vi "API Demo.vi"() -> ()   [LabVIEW 2020]
uses:
  Framework/Test Case/LUnit Test Case.lvclass
  Framework/Result Classes/Method Result/Method Result.lvclass/Method Result.ctl
  Framework/Result Classes/Test Case Result/Test Case Result.lvclass/Test Case Result.ctl
  Framework/Result Classes/Test Suite Result/Test Suite Result.lvclass/Test Suite Result.ctl
  Framework/Result Classes/Test Case Result/Private/SubVIs/Merge Status.vi
  Framework/Execution API/Execution API.lvclass
  Framework/Result Classes/Method Result/Method Result.lvclass
  Framework/Result Classes/Test Case Result/Test Case Result.lvclass
  Framework/Result Classes/Test Suite Result/Test Suite Result.lvclass
panel:
  in  "Tab Control":enum32{"Path", "Test Case", "App Instance"}(tab)
  in  "Project or Class Path":path
  in  "Class path":path
  out "error out":errorcluster
  in  "error in":errorcluster
  in  "Stop":bool
  out "Status":string
  # "1. Select which method you want to use for finding tests to run from the API by choosing a tab in the tab control.\n2. Fill in the path to the test to run. \n3. Run this VI."
  # "Enter the path to a test case class, lvlib or a project containing the test cases."
  # "Execute all tests found in the current application instance"
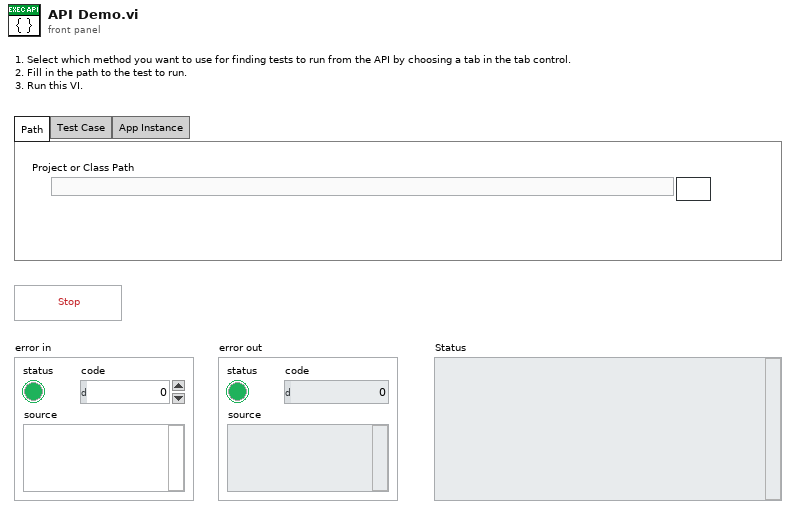
[diagram p1: front panel]
types:
  T1 = cluster{"Event Registration Refnum":refnum<event-registration>, "Event Registration Refnum":refnum<event-registration>}
  T2 = typedef "Assertion Result.lvclass/Status.ctl" = enum16{"Pass", "Fail", "Error", "Skipped", "Setup Error", "Broken", "Teardown Error"}
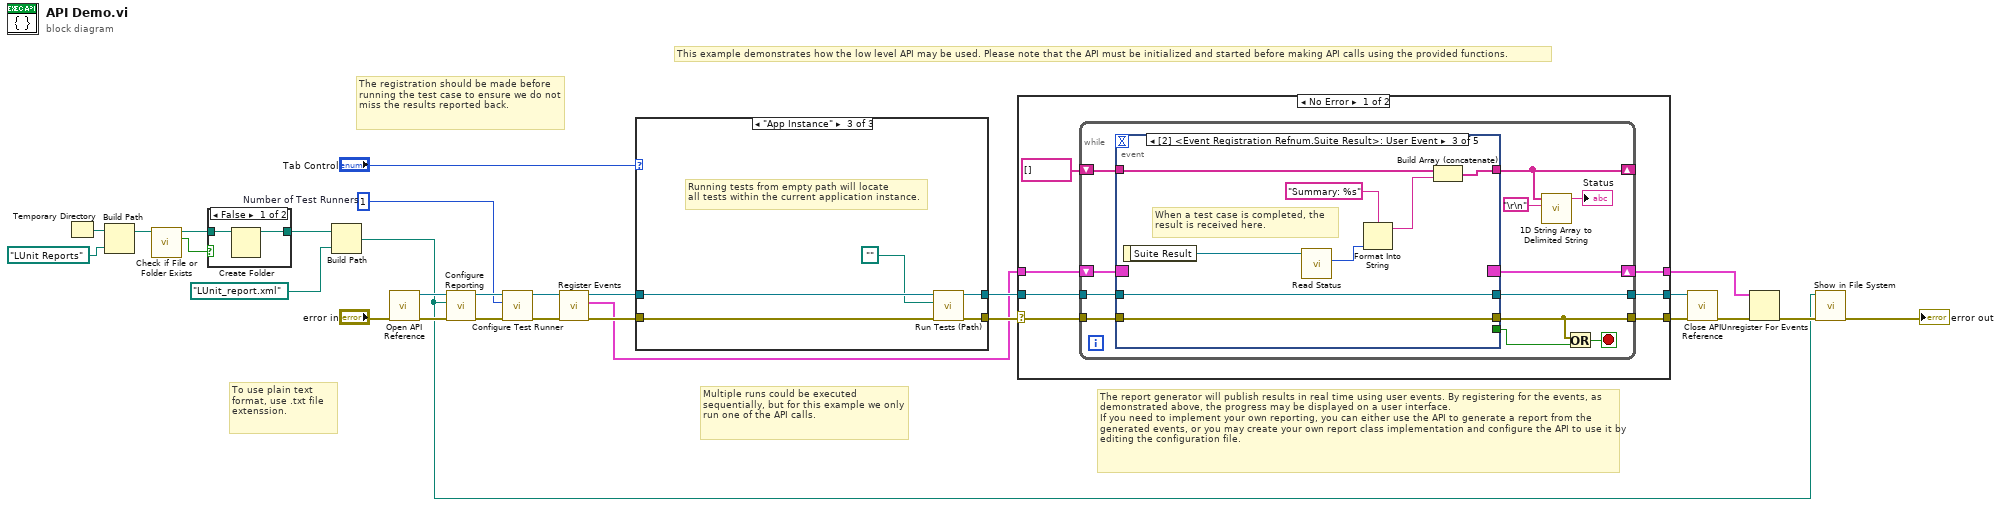
[diagram p0: block diagram]
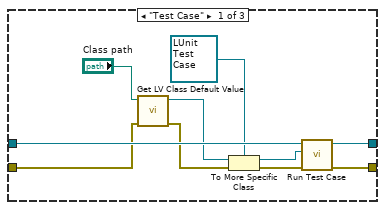
[diagram p3: hidden frame]
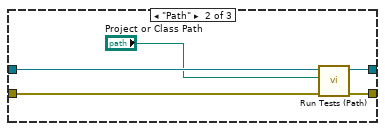
[diagram p4: hidden frame]
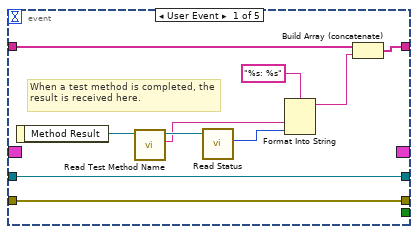
[diagram p5: hidden frame]
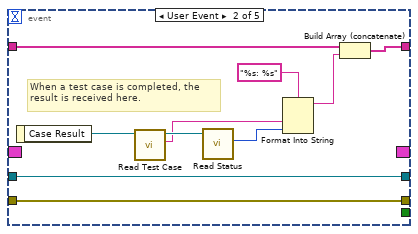
[diagram p6: hidden frame]
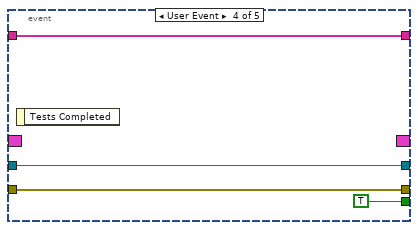
[diagram p7: hidden frame]
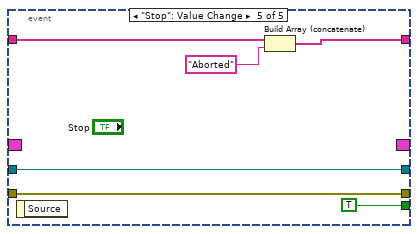
[diagram p8: hidden frame]
diagram:
  w11 = 1  # Number of Test Runners
  # "To use plain text format, use .txt file extenssion."
  # "The registration should be made before running the test case to ensure we do not miss the results reported back."
  # "The report generator will publish results in real time using user events. By registering for the events, as demonstrated above, the progress may be displayed on a user interface. \nIf you need to implement your own reporting, you can either use the API to generate a report from the generated events, or you may create your own report class implementation and configure the API to use it by editing the configuration file."
  # "This example demonstrates how the low level API may be used. Please note that the API must be initialized and started before making API calls using the provided functions."
  # "Multiple runs could be executed sequentially, but for this example we only run one of the API calls."
  n1 = Temporary Directory() -> (w5:path)
  n2 = Build Path(base path=w5, name or relative path=path "LUnit Reports") -> (appended path=w6:path)
  n3 = call <vilib>:"Check if File or Folder Exists.vi"("path"=w6) -> ("file or folder exists?"=w2:bool, "dup path"=w3:path)  [unwired: 8 in, 1 out]
  n4 = case shown="False" w2 {
    tunnel: w3 -> [w30 w31]
    tunnel: [w29 w31] -> w1
    frame False {
      n5 = Create Folder(path (use dialog)=w30) -> (created path=w29:path)  [unwired: 2 in, 2 out]
    }
    frame True {
    }
  }
  n6 = Build Path(base path=w1, name or relative path=path "LUnit_report.xml") -> (appended path=w7:path)
  n7 = call "Open API Reference.vi"("error in (no error)"="error in") -> ("error out"=w17:errorcluster, "Execution API out"=w13:refnum<class "Execution API.lvclass">)  [unwired: 9 in]
  n8 = call "Configure Reporting.vi"("error in (no error)"=w17, "Path"=w7, "Execution API In"=w13) -> ("error out"=w15:errorcluster, "Execution API Out"=w16:refnum<class "Execution API.lvclass">)  [unwired: 7 in]
  n9 = call "Configure Test Runner.vi"("error in (no error)"=w15, "Number of Test Runners"=w11, "Execution API In"=w16) -> ("error out"=w14:errorcluster, "Execution API Out"=w12:refnum<class "Execution API.lvclass">)  [unwired: 7 in]
  n10 = call "Register Events.vi"("error in (no error)"=w14, "Execution API In"=w12) -> ("error out"=w20:errorcluster, "Result Events"=w18:T1, "Execution API Out"=w19:refnum<class "Execution API.lvclass">)  [unwired: 7 in]
  n11 = case shown="\"App Instance\"" "Tab Control" {
    tunnel: w19 -> [w41 w46 w51]
    tunnel: w20 -> [w37 w45 w50]
    tunnel: [w39 w44 w49] -> w28
    tunnel: [w40 w43 w48] -> w27
    frame "Test Case" {
      n12 = call <vilib>:"Get LV Class Default Value.vi"("error in (no error)"=w37, "class path"="Class path") -> ("error out"=w35:errorcluster, "object"=w36:refnum<class>)  [unwired: 8 in]
      n13 = To More Specific Class(target class=refnum<class "LUnit Test Case.lvclass"> refnum ("Test Case.lvclass"), reference=w36, error in=w35) -> (specific class reference=w33:refnum<class "LUnit Test Case.lvclass">, error out=w34:errorcluster)
      n14 = call "Run Test Case.vi"("error in (no error)"=w34, "Test Case"=w33, "Execution API In"=w41) -> ("error out"=w40:errorcluster, "Execution API Out"=w39:refnum<class "Execution API.lvclass">)  [unwired: 7 in]
    }
    frame "Path" {
      n15 = call "Run Tests (Path).vi"("error in (no error)"=w45, "Project or Class Path"="Project or Class Path", "Execution API In"=w46) -> ("error out"=w43:errorcluster, "Execution API Out"=w44:refnum<class "Execution API.lvclass">)  [unwired: 7 in]
    }
    frame "App Instance" {
      # "Running tests from empty path will locate\nall tests within the current application instance."
      n16 = call "Run Tests (Path).vi"("error in (no error)"=w50, "Project or Class Path"=path "", "Execution API In"=w51) -> ("error out"=w48:errorcluster, "Execution API Out"=w49:refnum<class "Execution API.lvclass">)  [unwired: 7 in]
    }
  }
  n17 = case shown="No Error" w27 {
    selector: w27 -> [w57 w111]
    tunnel: w18 -> [w58 w109]
    tunnel: w28 -> [w56 w110]
    tunnel: [w54 w111] -> w26
    tunnel: [w53 w110] -> w25
    tunnel: [w52 w109] -> w22
    frame No Error {
      n18 = while {
        tunnel: w57 -> [w69]
        tunnel: w56 -> [w68]
        tunnel: [w66] -> w53
        tunnel: [w60] -> w54
        shift-right: [w62] -> _
        shift-left: string[] [] -> [w63]
        shift-right: [w59] -> w52
        shift-left: w58 -> [w70]
        stop <- w61 stop-if-true
        n19 = event shown="[2] <Event Registration Refnum.Suite Result>: User Event" {
          selector: w70 -> [_ _ _ _ _]
          dyn-events: [_ _ _ _ _] -> w59
          timeout: _ -> [_ _ _ _ _]
          tunnel: w69 -> [w71 w81 w91 w101 w107]
          tunnel: w68 -> [w80 w90 w98 w102 w108]
          tunnel: [_ _ _ TRUE TRUE] -> w67
          tunnel: [w80 w90 w98 w102 w108] -> w66
          tunnel: [w71 w81 w91 w101 w107] -> w60
          tunnel: w63 -> [w74 w84 w94 w99 w106]
          tunnel: [w73 w83 w93 w99 w105] -> w62
          event User Event {
            # "When a test method is completed, the result is received here."
            n20 = event-data() -> ("Method Result"=w79:refnum<class "Method Result.lvclass">)  [unwired: 1 in]
            n21 = call "Read Test Method Name.vi"("Method Result In"=w79) -> ("Test Method Name"=w77:string, "Method Result Out"=w78:refnum<class "Method Result.lvclass">)  [unwired: 9 in]
            n22 = call "Read Status.vi"("Method Result In"=w78) -> ("Status"=w76:T2)  [unwired: 8 in, 2 out]
            n23 = Format Into String(format string="%s: %s", w77, w76) -> (resulting string=w72:string)  [unwired: 2 in, 1 out]
            n24 = Build Array (concatenate)(w74, w72) -> (w73:string[])
          }
          event User Event {
            # "When a test case is completed, the result is received here."
            n25 = event-data() -> ("Case Result"=w89:refnum<class "Test Case Result.lvclass">)  [unwired: 1 in]
            n26 = call "Read Test Case.vi"("Test Case Result In"=w89) -> ("Test Case"=w87:string, "Test Case Result Out"=w88:refnum<class "Test Case Result.lvclass">)  [unwired: 9 in]
            n27 = call "Read Status.vi"("Test Case Result In"=w88) -> ("Status"=w86:T2)  [unwired: 8 in, 2 out]
            n28 = Format Into String(format string="%s: %s", w87, w86) -> (resulting string=w82:string)  [unwired: 2 in, 1 out]
            n29 = Build Array (concatenate)(w84, w82) -> (w83:string[])
          }
          event User Event {
            # "When a test case is completed, the result is received here."
            n30 = event-data() -> ("Suite Result"=w97:refnum<class "Test Suite Result.lvclass">)  [unwired: 1 in]
            n31 = call "Read Status.vi"("Test Suite Result In"=w97) -> ("Status"=w96:T2)  [unwired: 9 in, 1 out]
            n32 = Format Into String(format string="Summary: %s", w96) -> (resulting string=w92:string)  [unwired: 2 in, 1 out]
            n33 = Build Array (concatenate)(w94, w92) -> (w93:string[])
          }
          event User Event {
            n34 = event-data() -> ()  [unwired: 1 in, 1 out]
          }
          event "Stop": Value Change {
            n35 = event-data() -> ()  [unwired: 1 in, 1 out]
            n36 = Build Array (concatenate)(w106, "Aborted") -> (w105:string[])
          }
        }
        n37 = call <vilib>:"1D String Array to Delimited String.vi"("delimiter"="\r\n", "string array"=w62) -> ("delimited string"=→"Status":string)  [unwired: 9 in]
        n38 = Or(x=w60, y=w67) -> (x .or. y?=w61:bool)
      }
    }
    frame Error {
    }
  }
  n39 = call "Close API Reference.vi"("error in (no error)"=w26, "Execution API in"=w25) -> ("error out"=w21:errorcluster)  [unwired: 9 in]
  n40 = Unregister For Events(event registration refnum=w22, error in=w21) -> (error out=w9:errorcluster)
  n41 = call <vilib>:"Show in File System.vi"("error in (no error)"=w9, "file or directory path"=w7) -> ("error out"=→"error out":errorcluster)  [unwired: 9 in]
